vi "MSBH_MSBL.vi"(11 "Hex Array Out":string[](array[string])) -> (3 "Value":u32)   [LabVIEW 2016]
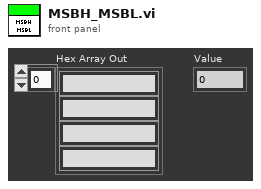
[diagram p1: front panel]
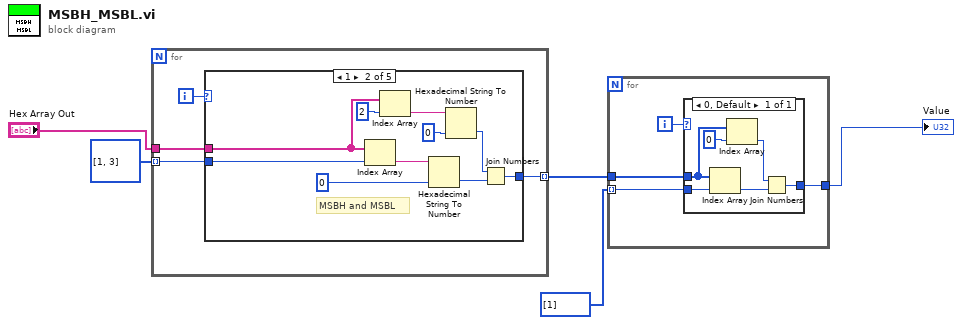
[diagram p0: block diagram]
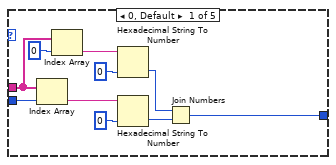
[diagram p2: hidden frame]
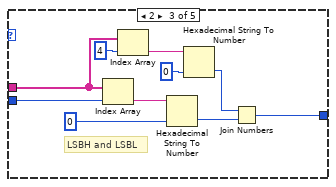
[diagram p3: hidden frame]
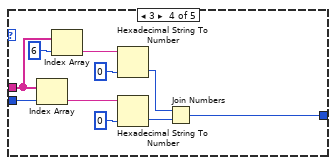
[diagram p4: hidden frame]
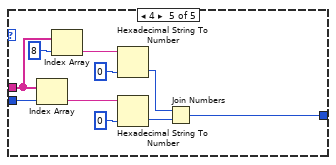
[diagram p5: hidden frame]
diagram:
  n1 = for {
    tunnel: "Hex Array Out" -> [w9]
    tunnel: u8[] [1, 3] -> [w8] mode=indexing
    tunnel: [w6] -> w3 mode=indexing
    i -> [w7]
    n2 = case shown="1" w7 {
      tunnel: w9 -> [w14 w25 w32 w42 w52]
      tunnel: w8 -> [w13 w24 w31 w40 w51]
      tunnel: [w17 w20 w30 w41 w50] -> w6
      frame 0, Default {
        n3 = Index Array(array=w14, index=w13) -> (element=w12:string)
        n4 = Index Array(array=w14, index=0) -> (element=w16:string)
        n5 = Hexadecimal String To Number(string=w16, default (0uL)=u8 0 ("default (0 U32)")) -> (number=w19:u8)  [unwired: 1 in, 1 out]
        n6 = Hexadecimal String To Number(string=w12, default (0uL)=u8 0 ("default (0 U32)")) -> (number=w10:u8)  [unwired: 1 in, 1 out]
        n7 = Join Numbers(hi=w19, lo=w10) -> ((hi.lo)=w17:u16)
      }
      frame 1 {
        # "MSBH and MSBL"
        n8 = Index Array(array=w25, index=w24) -> (element=w23:string)
        n9 = Index Array(array=w25, index=2) -> (element=w26:string)
        n10 = Hexadecimal String To Number(string=w23, default (0uL)=u8 0 ("default (0 U32)")) -> (number=w21:u8)  [unwired: 1 in, 1 out]
        n11 = Hexadecimal String To Number(string=w26, default (0uL)=u8 0 ("default (0 U32)")) -> (number=w29:u8)  [unwired: 1 in, 1 out]
        n12 = Join Numbers(hi=w29, lo=w21) -> ((hi.lo)=w20:u16)
      }
      frame 2 {
        # "LSBH and LSBL"
        n13 = Index Array(array=w32, index=w31) -> (element=w35:string)
        n14 = Index Array(array=w32, index=4) -> (element=w36:string)
        n15 = Hexadecimal String To Number(string=w35, default (0uL)=u8 0 ("default (0 U32)")) -> (number=w33:u8)  [unwired: 1 in, 1 out]
        n16 = Hexadecimal String To Number(string=w36, default (0uL)=u8 0 ("default (0 U32)")) -> (number=w39:u8)  [unwired: 1 in, 1 out]
        n17 = Join Numbers(hi=w39, lo=w33) -> ((hi.lo)=w30:u16)
      }
      frame 3 {
        n18 = Index Array(array=w42, index=w40) -> (element=w45:string)
        n19 = Index Array(array=w42, index=6) -> (element=w46:string)
        n20 = Hexadecimal String To Number(string=w46, default (0uL)=u8 0 ("default (0 U32)")) -> (number=w49:u8)  [unwired: 1 in, 1 out]
        n21 = Hexadecimal String To Number(string=w45, default (0uL)=u8 0 ("default (0 U32)")) -> (number=w43:u8)  [unwired: 1 in, 1 out]
        n22 = Join Numbers(hi=w49, lo=w43) -> ((hi.lo)=w41:u16)
      }
      frame 4 {
        n23 = Index Array(array=w52, index=w51) -> (element=w55:string)
        n24 = Index Array(array=w52, index=8) -> (element=w56:string)
        n25 = Hexadecimal String To Number(string=w56, default (0uL)=u8 0 ("default (0 U32)")) -> (number=w59:u8)  [unwired: 1 in, 1 out]
        n26 = Hexadecimal String To Number(string=w55, default (0uL)=u8 0 ("default (0 U32)")) -> (number=w53:u8)  [unwired: 1 in, 1 out]
        n27 = Join Numbers(hi=w59, lo=w53) -> ((hi.lo)=w50:u16)
      }
    }
  }
  n28 = for {
    tunnel: w3 -> [w62]
    tunnel: u8[] [1] -> [w61] mode=indexing
    tunnel: [w60] -> w5
    i -> [w63]
    n29 = case shown="0, Default" w63 {
      tunnel: w62 -> [w65]
      tunnel: w61 -> [w66]
      tunnel: [w67] -> w60
      frame 0, Default {
        n30 = Index Array(array=w65, index=w66) -> (element=w64:u16)
        n31 = Index Array(array=w65, index=0) -> (element=w69:u16)
        n32 = Join Numbers(hi=w69, lo=w64) -> ((hi.lo)=w67:u32)
      }
    }
  }
  "Value" <- w5
